vi "RSNRPZ Set Result Update Time.vi"(8 "error in (no error)":errorcluster, 9 "Result Update Time (0.1 s)":dbl=0.1 format="%^.3e", 10 "Channel (1)":i32=1, 11 "VISA session":refnum<visa-resource-name> caption="VISA resource name") -> (0 "error out":errorcluster, 3 "dup VISA session":refnum<visa-resource-name> caption="VISA resource name")   [LabVIEW 2010]
doc: "This VI sets result update time, which influences USB traffic if sensor is in continuous sweep mode.\n\nNote:\n\n1) This VI is available only for NRP-Z81.\n\nRemote-control command(s):\nSYST:RUT"
uses:
  rsnrpz_32.dll
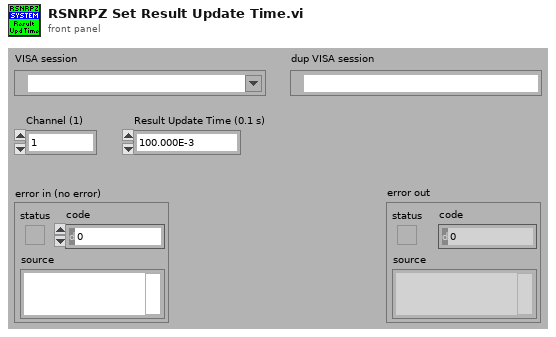
[diagram p1: front panel]
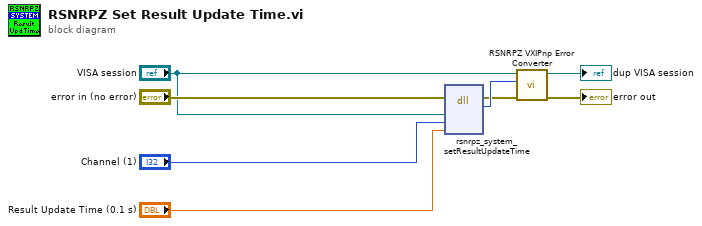
[diagram p0: block diagram]
diagram:
  n1 = dll-call lib="rsnrpz_32.dll" fn="rsnrpz_system_setResultUpdateTime"(error in="error in (no error)", "Instrument Handle"="VISA session", "Channel"="Channel (1)", "Result Update Time"="Result Update Time (0.1 s)") -> (error out=w5:errorcluster, "Status"=w8:i32)  [unwired: 5 in, 1 out]
  n2 = call <instrlib>:"RSNRPZ VXIPnp Error Converter.vi"("error in"=w5, "VXIPnp error code"=w8, "VISA session"="VISA session") -> ("error out"=→"error out":errorcluster, "dup VISA session"=→"dup VISA session":refnum<visa-resource-name>)  [unwired: 7 in]
